vi "Generate Custom Trace.vi"(8 "error in (no error)":errorcluster, 10 "Custom Action":string) -> ()   [LabVIEW 2020, in "AF Debug.lvlib"]
doc: "<p>Generates a DETT (Desktop Execution Trace Toolkit) User Generated Trace. The trace includes the source actor's ID (or debug alias, if available) and a custom message you define.</p>"
uses:
  AF Debug.lvlib
  ActorFramework/Actor Framework.lvlib
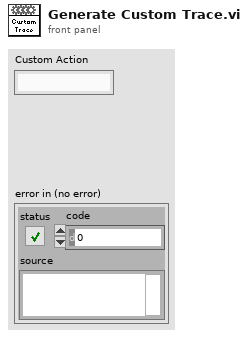
[diagram p1: front panel]
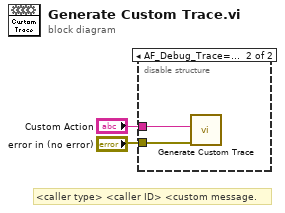
[diagram p0: block diagram]
diagram:
  # "<caller type> <caller ID> <custom message."
  n1 = disable-structure shown="AF_Debug_Trace==TRUE" {
    disable-tunnel: "Custom Action" -> [_ w3]
    disable-tunnel: "error in (no error)" -> [_ w4]
    frame condition #0 {
    }
    frame condition #1 (active) {
      n2 = call "Generate Custom Trace.vi"("error in (no error)"=w4, "Custom Action"=w3) -> ()  [unwired: 10 in]
    }
  }
